vi "TMYTEK_BBox_Ctrl.vi"() -> ()   [LabVIEW 2019]
uses:
  <vilib>/FPGAPlugInAG/USRP 294xR; 295xR 120 MSps/niLvFpga_Open_USRP 294xR; 295xR 120 MSps.vi
  <vilib>/rvi/interface/common/dynamic/niFpgaDynamicAddResources.vi
  <vilib>/Utility/error.llb/Error Cluster From Error Code.vi
  <vilib>/rvi/errors/niLvFpgaAdjustHostInterfaceError.vi
  <vilib>/FPGAPlugInAG/Dynamic/niLvFpga_Close_Dynamic.vi
  <vilib>/rvi/interface/nirviOpenFPGA/nirviOpenFPGA.xnode
  FPGA Bitfiles/spi_FPGATarget_FPGAMain_AAR7OmfWQ-g.lvbitx
  FPGA/TMYTEK_FPGA_Ctrl.vi
  <vilib>/rvi/interface/nirviReadWriteControl/nirviReadWriteControl.xnode
  <vilib>/rvi/interface/nirviMethod/nirviMethod.xnode
  <vilib>/rvi/interface/nirviCloseFPGA/nirviCloseFPGA.xnode
  NiFpgaLv.dll
  <vilib>/rvi/interface/Simulation/niFpgaSimulationCallBeginRW.vi
  <vilib>/FPGAPlugInAG/Dynamic/niLvFpga_WriteFifo_Dynamic.vi
  <vilib>/rvi/errors/niLvFpgaMergeErrorWithErrorCode.vi
panel:
  out "String":string
  in  "Delay Step":u16=9
  in  "Mode":T1(ring)
  in  "Write":bool
  in  "Index":u8 format="%06b"
  in  "Ctrl Pattern":u8 format="%03b"
  in  "Ctrl Pattern":u8 format="%04b"
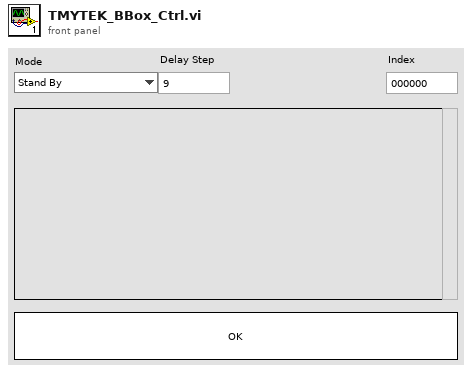
[diagram p1: front panel]
types:
  T1 = enum16{"Stand By", "Tx Mode", "Rx Mode", "Sleep"}
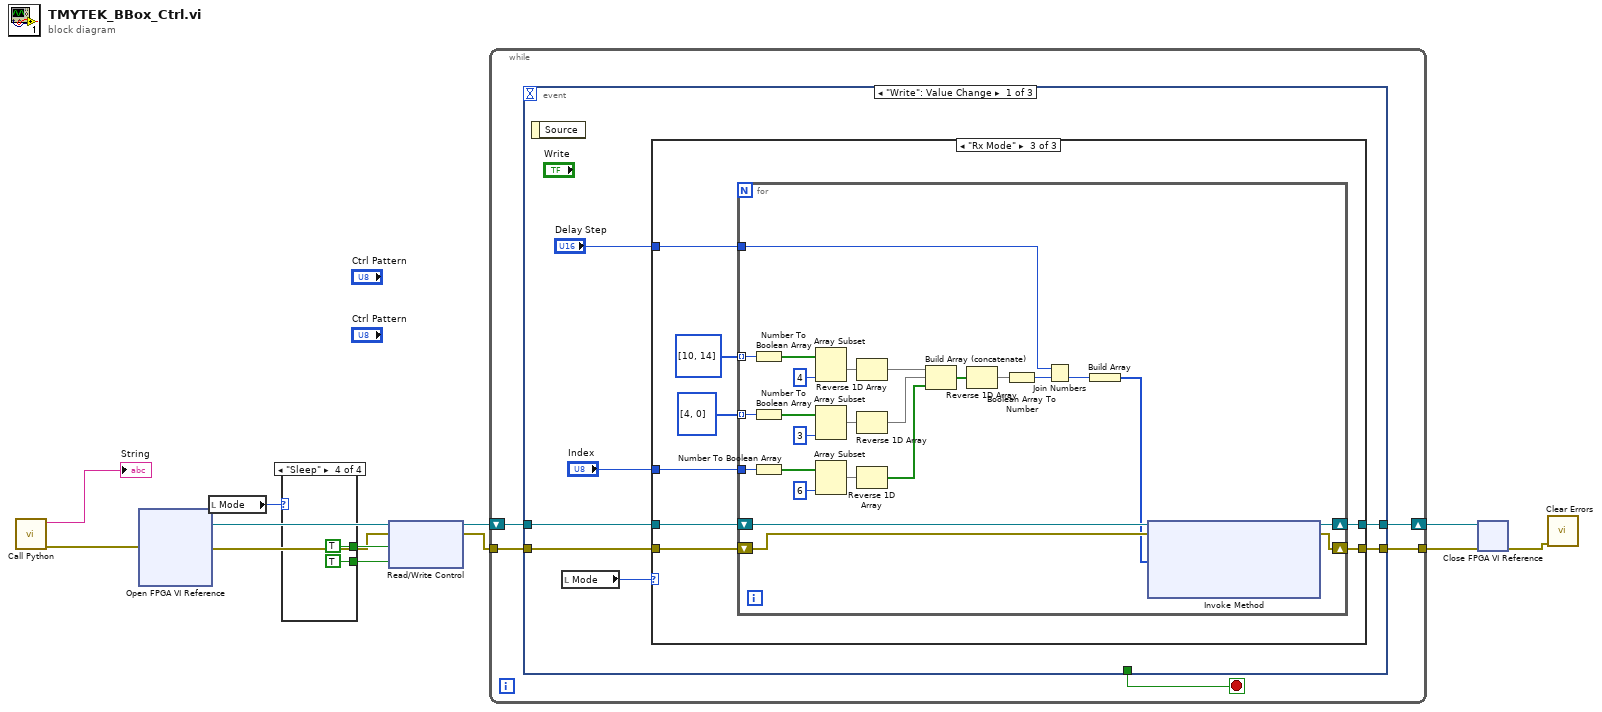
[diagram p0: block diagram]
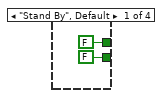
[diagram p2: hidden frame]
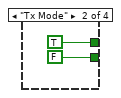
[diagram p3: hidden frame]
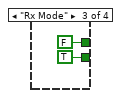
[diagram p4: hidden frame]
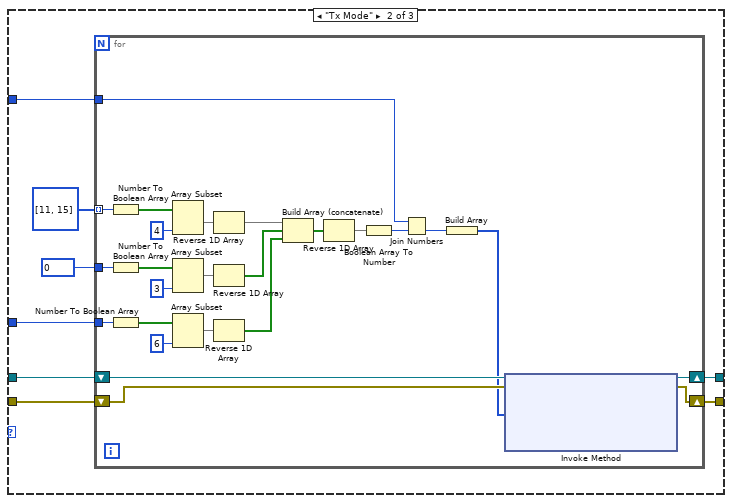
[diagram p6: hidden frame]
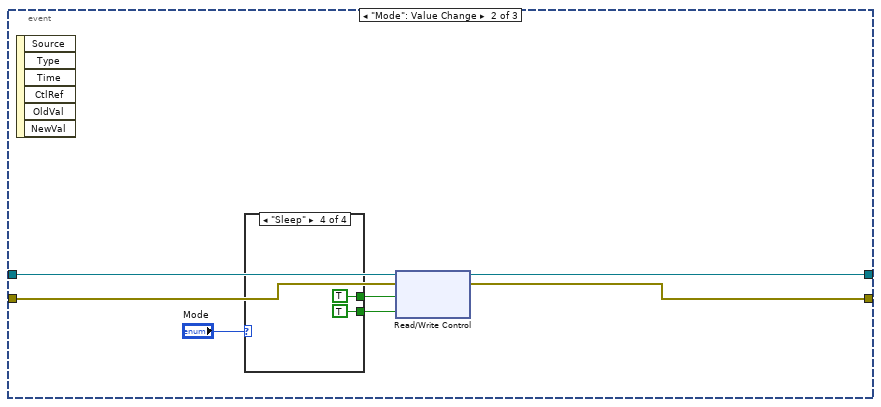
[diagram p7: hidden frame]
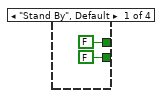
[diagram p8: hidden frame]
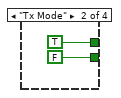
[diagram p9: hidden frame]
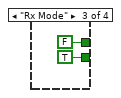
[diagram p10: hidden frame]
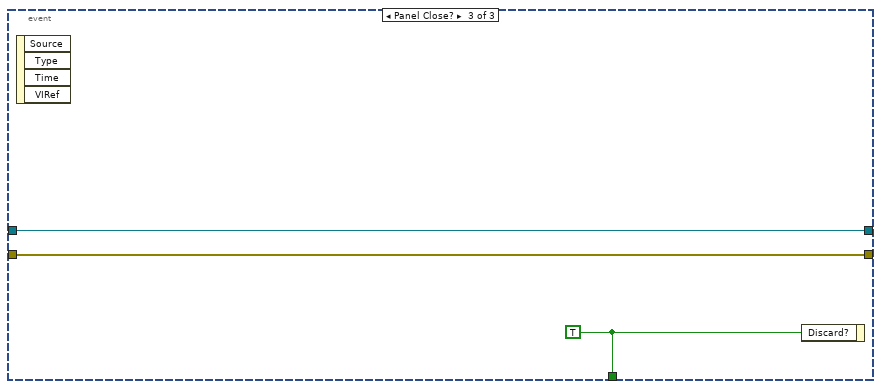
[diagram p11: hidden frame]
diagram:
  n1 = call "Call Python.vi"() -> ("error out"=w2:errorcluster, "String"=→"String":string)  [unwired: 10 in]
  n2 = xnode "Open FPGA VI Reference"("error in"=w2) -> ("FPGA VI Reference Out"=w8:refnum<k20>, "error out"=w7:errorcluster)  [unwired: 1 in]
  n3 = local read "Mode"() -> (w4:T1)
  n4 = case shown="\"Sleep\"" w4 {
    tunnel: [FALSE TRUE FALSE TRUE] -> w9
    tunnel: [FALSE FALSE TRUE TRUE] -> w10
    frame "Stand By", Default {
    }
    frame "Tx Mode" {
    }
    frame "Rx Mode" {
    }
    frame "Sleep" {
    }
  }
  n5 = xnode "Read/Write Control"("FPGA VI Reference In"=w8, "error in"=w7, "AUX I/O 6"=w9, "AUX I/O 7"=w10) -> ("FPGA VI Reference Out"=w6:refnum<k20>, "error out"=w5:errorcluster)
  n6 = while {
    tunnel: w5 -> [w24]
    shift-right: [w23] -> w12
    shift-left: w6 -> [w25]
    tunnel: [w21] -> w11
    stop <- w22 stop-if-true
    n7 = event shown="[0] \"Write\": Value Change" {
      selector: _ -> [_ _ _]
      dyn-events: _ -> [_ _ _]
      timeout: _ -> [_ _ _]
      tunnel: w25 -> [w32 w107 w117]
      tunnel: w24 -> [w31 w106 w116]
      tunnel: [w30 w105 w117] -> w23
      tunnel: [_ _ w118] -> w22
      tunnel: [w29 w104 w116] -> w21
      event "Write": Value Change {
        n8 = event-data() -> ()  [unwired: 1 in, 1 out]
        n9 = local read "Mode"() -> (w26:T1)
        n10 = case shown="\"Rx Mode\"" w26 {
          tunnel: w32 -> [w34 w42 w75]
          tunnel: w31 -> [w33 w41 w74]
          tunnel: [w34 w40 w73] -> w30
          tunnel: [w33 w39 w72] -> w29
          tunnel: "Index" -> [_ w38 w71]
          tunnel: "Delay Step" -> [_ w36 w70]
          frame Default {
          }
          frame "Tx Mode" {
            n11 = for {
              tunnel: w38 -> [w52]
              tunnel: u8 0 ("Ctrl Pattern 2") -> [w51]
              tunnel: u8[] [11, 15] -> [w50] mode=indexing
              tunnel: w36 -> [w43]
              shift-right: [w65] -> w40
              shift-left: w42 -> [w67]
              shift-right: [w64] -> w39
              shift-left: w41 -> [w66]
              n12 = Number To Boolean Array(number=w50) -> (Boolean array=w54:bool[])
              n13 = Number To Boolean Array(number=w51) -> (Boolean array=w55:bool[])
              n14 = Number To Boolean Array(number=w52) -> (Boolean array=w56:bool[])
              n15 = Array Subset(array=w54, length=4) -> (w53:bool[])  [unwired: 1 in]
              n16 = Array Subset(array=w55, length=3) -> (w58:bool[])  [unwired: 1 in]
              n17 = Array Subset(array=w56, length=6) -> (w57:bool[])  [unwired: 1 in]
              n18 = Reverse 1D Array(array=w53) -> (reversed array=w59:bool[])
              n19 = Reverse 1D Array(array=w58) -> (reversed array=w60:bool[])
              n20 = Reverse 1D Array(array=w57) -> (reversed array=w61:bool[])
              n21 = Build Array (concatenate)(w59, w60, w61) -> (w62:bool[])
              n22 = Reverse 1D Array(array=w62) -> (reversed array=w63:bool[])
              n23 = Boolean Array To Number(Boolean array=w63) -> (number=w46:u16)
              n24 = Join Numbers(hi=w43, lo=w46) -> ((hi.lo)=w44:u32)
              n25 = Build Array(w44) -> (w45:u32[])
              n26 = xnode "Invoke Method"("FPGA VI Reference In"=w67, "error in"=w66, "Data"=w45) -> ("FPGA VI Reference Out"=w65:refnum<k20>, "error out"=w64:errorcluster)  [unwired: 1 in, 1 out]
            }
          }
          frame "Rx Mode" {
            n27 = for {
              tunnel: w71 -> [w85]
              tunnel: u8[] [4, 0] -> [w84] mode=indexing
              tunnel: u8[] [10, 14] -> [w83] mode=indexing
              tunnel: w70 -> [w76]
              shift-right: [w98] -> w73
              shift-left: w75 -> [w100]
              shift-right: [w97] -> w72
              shift-left: w74 -> [w99]
              n28 = Number To Boolean Array(number=w83) -> (Boolean array=w87:bool[])
              n29 = Number To Boolean Array(number=w84) -> (Boolean array=w88:bool[])
              n30 = Number To Boolean Array(number=w85) -> (Boolean array=w89:bool[])
              n31 = Array Subset(array=w87, length=4) -> (w86:bool[])  [unwired: 1 in]
              n32 = Array Subset(array=w88, length=3) -> (w91:bool[])  [unwired: 1 in]
              n33 = Array Subset(array=w89, length=6) -> (w90:bool[])  [unwired: 1 in]
              n34 = Reverse 1D Array(array=w86) -> (reversed array=w92:bool[])
              n35 = Reverse 1D Array(array=w91) -> (reversed array=w93:bool[])
              n36 = Reverse 1D Array(array=w90) -> (reversed array=w94:bool[])
              n37 = Build Array (concatenate)(w92, w93, w94) -> (w95:bool[])
              n38 = Reverse 1D Array(array=w95) -> (reversed array=w96:bool[])
              n39 = Boolean Array To Number(Boolean array=w96) -> (number=w79:u16)
              n40 = Join Numbers(hi=w76, lo=w79) -> ((hi.lo)=w77:u32)
              n41 = Build Array(w77) -> (w78:u32[])
              n42 = xnode "Invoke Method"("FPGA VI Reference In"=w100, "error in"=w99, "Data"=w78) -> ("FPGA VI Reference Out"=w98:refnum<k20>, "error out"=w97:errorcluster)  [unwired: 1 in, 1 out]
            }
          }
        }
      }
      event "Mode": Value Change {
        n43 = event-data() -> ()  [unwired: 1 in, 6 out]
        n44 = case shown="\"Sleep\"" "Mode" {
          tunnel: [FALSE TRUE FALSE TRUE] -> w102
          tunnel: [FALSE FALSE TRUE TRUE] -> w101
          frame "Stand By", Default {
          }
          frame "Tx Mode" {
          }
          frame "Rx Mode" {
          }
          frame "Sleep" {
          }
        }
        n45 = xnode "Read/Write Control"("FPGA VI Reference In"=w107, "error in"=w106, "AUX I/O 6"=w102, "AUX I/O 7"=w101) -> ("FPGA VI Reference Out"=w105:refnum<k20>, "error out"=w104:errorcluster)
      }
      event Panel Close? {
        w118 = TRUE ("Discard?")
        n46 = event-data() -> ()  [unwired: 1 in, 4 out]
        n47 = event-data("Discard?"=w118) -> ()  [unwired: 1 in, 1 out]
      }
    }
  }
  n48 = xnode "Close FPGA VI Reference"("FPGA VI Reference In"=w12, "error in"=w11) -> ("error out"=w3:errorcluster)
  n49 = call <vilib>:"Clear Errors.vi"("error in (no error)"=w3) -> ()  [unwired: 5 in, 2 out]
